vi "1D Time Stamp.vi"(4 "column vector (F)":bool, 5 "format string":string="%Y-%m-%dT%H:%M:%S%20u", 7 "key description":string, 8 "sections":string[](array[string]), 9 "time stamp":timestamp[](array[timestamp]), 11 "info data":string) -> (0 "sections out":string[](array[string]), 3 "info data out":string)   [LabVIEW 2013, in "infolib.lvlib"]
doc: "Add a new new date and time table to Info Data string. If section exists in Info Data string, inserts key into this section."
uses:
  infolib.lvlib
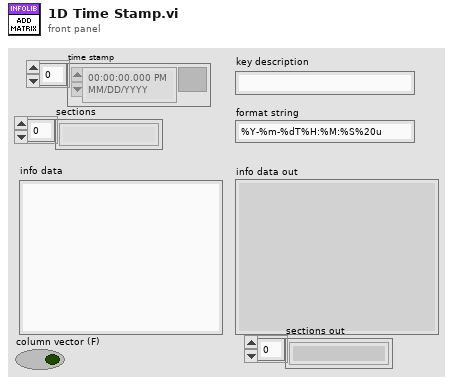
[diagram p1: front panel]
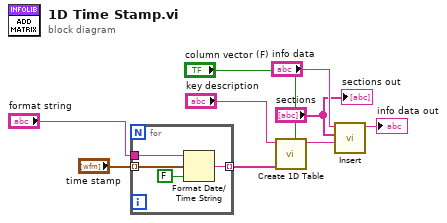
[diagram p0: block diagram]
diagram:
  n1 = for {
    tunnel: "format string" -> [w12]
    tunnel: "time stamp" -> [w13] mode=indexing
    tunnel: [w11] -> w4 mode=indexing
    n2 = Format Date/Time String(time format string (%c)=w12, seconds (now)=w13, UTC format=FALSE) -> (date/time string=w11:string)
  }
  n3 = call "Create 1D Table.vi"("column vector (F)"="column vector (F)", "formatted values"=w4, "table name"="key description") -> ("table"=w2:string)  [unwired: 7 in, 1 out]
  n4 = call "Insert.vi"("insert"=w2, "sections"="sections", "info data"="info data") -> ("info data out"=→"info data out":string)  [unwired: 8 in]
  "sections out" <- "sections"
